vi "LTVDiffDriveCtrl_Execute_TrajState.vi"(5 "LTV_DiffDriveCtrl_Model":T5={"Track Width"=0.2, "Diff_Drive_Linear_System"={"m_A"=[], "m_B"=[], "m_C"=[], "m_D"=[], "States"=0, "Inputs"=0, "Outputs"=0}, "LTV_DiffDriveCtrl_Control"={"Max left vel ctrl effort V"=12.0, "Desired Heading Ctrl Tol Rad"=0.06, "Desired Y Pos Meas Tol M"=0.125, "Desired X Pos Ctrl Tol M"=0.125, "Desired Left Vel Ctrl Tol M/S"=0.1, "Desired Right Vel Ctrl Tol M/S"=0.1, "Max right vel ctrl effort V"=12.0}, "LTV_DiffDriveCtrl_Tolerance"={"Max Heading Tolerance Rad"=0.2, "Max X Tolerance M"=0.0625, "Max Y Tolerance M"=0.125, "Max Left Vel Tol M/S"=0.2, "Max Right Vel Tol M/S"=0.2}, "dT Sec"=0.02} {"LTV_DiffDriveCtrl_Tolerance"."Max Right Vel Tol M/S" format="%#_13g"; "LTV_DiffDriveCtrl_Tolerance"."Max Left Vel Tol M/S" format="%#_13g"; "LTV_DiffDriveCtrl_Tolerance"."Max Y Tolerance M" format="%#_13g"; "LTV_DiffDriveCtrl_Tolerance"."Max X Tolerance M" format="%#_13g"; "LTV_DiffDriveCtrl_Tolerance"."Max Heading Tolerance Rad" format="%#_13g"; "LTV_DiffDriveCtrl_Control"."Max right vel ctrl effort V" format="%#_13g"; "LTV_DiffDriveCtrl_Control"."Desired Right Vel Ctrl Tol M/S" format="%#_13g"; "LTV_DiffDriveCtrl_Control"."Desired Left Vel Ctrl Tol M/S" format="%#_13g"; "LTV_DiffDriveCtrl_Control"."Desired X Pos Ctrl Tol M" format="%#_13g"; "LTV_DiffDriveCtrl_Control"."Desired Y Pos Meas Tol M" format="%#_13g"; "LTV_DiffDriveCtrl_Control"."Desired Heading Ctrl Tol Rad" format="%#_13g"; "LTV_DiffDriveCtrl_Control"."Max left vel ctrl effort V" format="%#_13g"; "Track Width" format="%#_13g"}, 8 "Right Velocity":dbl, 9 "Left Velocity":dbl, 10 "CurrentPose":T2={"TRANSLATION"={"X"=0.0, "Y"=0.0}, "ROTATION"={"VALUE"=0.0, "COS"=1.0, "SIN"=0.0}} {"ROTATION"."SIN" format="%13.4f"; "ROTATION"."COS" format="%13.4f"; "ROTATION"."VALUE" format="%13.4f"; "TRANSLATION"."Y" format="%14.3f"; "TRANSLATION"."X" format="%14.3f"}, 11 "TRAJ_STATE":T1={"TimeSeconds"=0.0, "Velocity"=0.0, "Acceleration"=0.0, "POSE"={"TRANSLATION"={"X"=0.0, "Y"=0.0}, "ROTATION"={"VALUE"=0.0, "COS"=1.0, "SIN"=0.0}}, "Curvature"=0.0} {"POSE"."ROTATION"."SIN" format="%13.4f"; "POSE"."ROTATION"."COS" format="%13.4f"; "POSE"."ROTATION"."VALUE" format="%13.4f"; "POSE"."TRANSLATION"."Y" format="%14.3f"; "POSE"."TRANSLATION"."X" format="%14.3f"}) -> (0 "Error":bool, 1 "At Reference":bool, 2 "Right Motor Dmd":dbl, 3 "Left Motor Dmd":dbl, 4 "out LTV_DiffDrive_CONTROLLER":T10)   [LabVIEW 2019, in "Trajectory_Library.lvlib"]
doc: "The linear time-varying (LTV) differential drive controller has a similar form to the LQR, but the model used to compute the controller gain is the nonlinear model linearized around the drivetrain's current state. We precomputed gains for important places in our state-space, then interpolated between them with a look up table (LUT) to save computational resources.Filters the provided voltages to limit a differential drive's linear and angular acceleration.\n\nThis LabVIEW single call function creates and executes the LTV Diff Drive controller. \n\nThe input linear system is defined as:\n - states\n - left velocity (m/s)\n - right velocity (m/s)\n - inputs\n - left voltage (volts)\n - right voltage(volts)\n - outputs\n - left velocity (m/s)\n - right velocity (m/s)\n\n\n\nInputs:\n - LTVDiffDriveCtrl Model -- cluster -- Packed data used to construct the LTV Diff Drive control system.\n - Traj state -- Traj state -- The desired trajectory state. Contains desired position and velocity values. (Meters, radians)\n - Ref Left Velocity -- double -- The desired left velocity (Meters/sec)\n - Ref Right Velocity -- double -- The desired right velocity (Meters/sec)\n - Current Pose -- Pose2d -- The current pose. (Meters, Radians)\n - Left Velocity -- double -- The current left velocity (Meters/sec)\n - Right Velocity -- double -- The current right velocity (Meters/sec)\n\nOutputs:\n - Left Motor Dmd -- double -- Left wheel motor demand (+/- 1.0)\n - Right Motor Dmd -- double -- Left wheel motor demand (+/- 1.0)\n - At Reference -- boolean -- If TRUE, the current position is within the tolerance.\n - Error -- boolean -- If TRUE, an error occured.\n - out LTV DiffDriveCtrl -- cluster -- Internal data structure."
uses:
  Trajectory_Library.lvlib
  TypeDef/LTV_DIFF_DRIVE_CTRL.ctl
  TypeDef/FUNCTION_GENERATOR_MATRIX.ctl
  <vilib>/Analysis/Matrix/Datatypes/RealMatrix.ctl
  TypeDef/POSE2D.ctl
  TypeDef/TRANSLATION2D.ctl
  TypeDef/ROTATION2D.ctl
  TypeDef/LTV_DIFF_DRIVE_CTRL_MODEL_PARAMS.CTL
  TypeDef/LINEAR_SYSTEM.ctl
  TypeDef/LTV_DIFF_DRIVE_CTRL_CONTROL_PARAMS.CTL
  TypeDef/LTV_DIFF_DRIVE_CTRL_TOLERANCE.CTL
  TypeDef/TRAJ_STATE.ctl
  <vilib>/Analysis/Matrix/NI_Matrix.lvlib
panel:
  # "<States,States>"
  # "<States,Inputs>"
  # "<Outputs,States>"
  # "<Outputs,Inputs>"
  # "< 5, 1 >"
  # "< 2, 1 >"
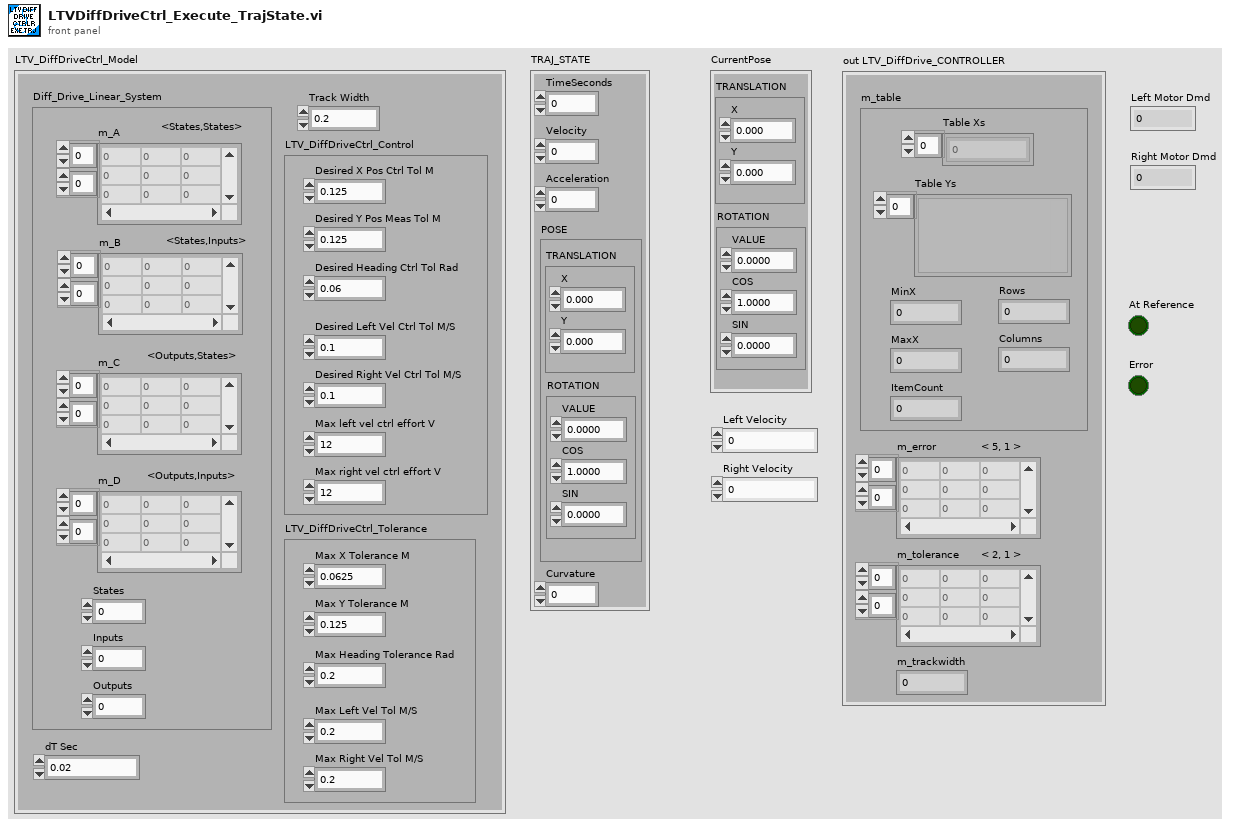
[diagram p1: front panel]
types:
  T1 = typedef "Trajectory_Library.lvlib/TRAJ_STATE.ctl" = cluster{"TimeSeconds":dbl, "Velocity":dbl, "Acceleration":dbl, "POSE":T2, "Curvature":dbl}
  T2 = typedef "Trajectory_Library.lvlib/POSE2D.ctl" = cluster{"TRANSLATION":T3, "ROTATION":T4}
  T3 = typedef "Trajectory_Library.lvlib/TRANSLATION2D.ctl" = cluster{"X":dbl, "Y":dbl}
  T4 = typedef "Trajectory_Library.lvlib/ROTATION2D.ctl" = cluster{"VALUE":dbl, "COS":dbl, "SIN":dbl}
  T5 = typedef "Trajectory_Library.lvlib/LTV_DIFF_DRIVE_CTRL_MODEL_PARAMS.CTL" = cluster{"Track Width":dbl, "Diff_Drive_Linear_System":T6, "LTV_DiffDriveCtrl_Control":T8, "LTV_DiffDriveCtrl_Tolerance":T9, "dT Sec":dbl}
  T6 = typedef "Trajectory_Library.lvlib/LINEAR_SYSTEM.ctl" = cluster{"m_A":T7, "m_B":T7, "m_C":T7, "m_D":T7, "States":i32, "Inputs":i32, "Outputs":i32}
  T7 = typedef "NI_Matrix.lvlib/RealMatrix.ctl" = dbl[][]
  T8 = typedef "Trajectory_Library.lvlib/LTV_DIFF_DRIVE_CTRL_CONTROL_PARAMS.CTL" = cluster{"Max left vel ctrl effort V":dbl, "Desired Heading Ctrl Tol Rad":dbl, "Desired Y Pos Meas Tol M":dbl, "Desired X Pos Ctrl Tol M":dbl, "Desired Left Vel Ctrl Tol M/S":dbl, "Desired Right Vel Ctrl Tol M/S":dbl, "Max right vel ctrl effort V":dbl}
  T9 = typedef "Trajectory_Library.lvlib/LTV_DIFF_DRIVE_CTRL_TOLERANCE.CTL" = cluster{"Max Heading Tolerance Rad":dbl, "Max X Tolerance M":dbl, "Max Y Tolerance M":dbl, "Max Left Vel Tol M/S":dbl, "Max Right Vel Tol M/S":dbl}
  T10 = typedef "Trajectory_Library.lvlib/LTV_DIFF_DRIVE_CTRL.ctl" = cluster{"m_table":T11, "m_error":T7, "m_tolerance":T7, "m_trackwidth":dbl}
  T11 = typedef "Trajectory_Library.lvlib/FUNCTION_GENERATOR_MATRIX.ctl" = cluster{"Table Xs":dbl[], "Table Ys":variant[], "MinX":dbl, "MaxX":dbl, "ItemCount":i32, "Rows":i32, "Columns":i32}
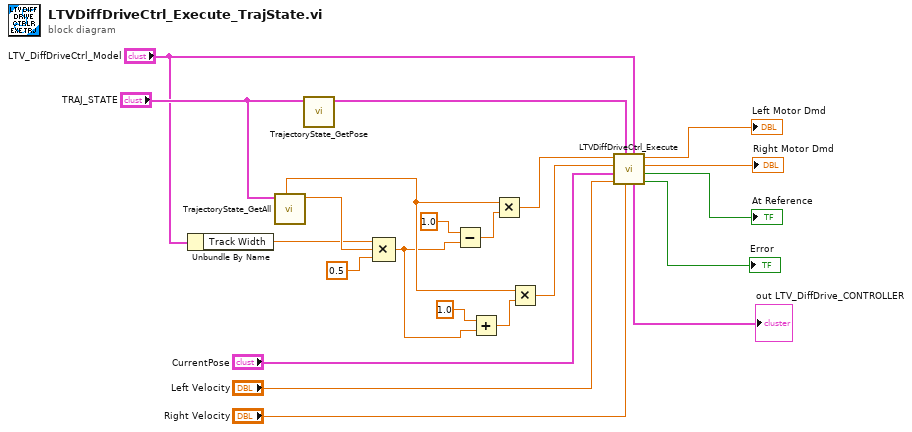
[diagram p0: block diagram]
diagram:
  n1 = Unbundle By Name("LTV_DiffDriveCtrl_Model") -> ("Track Width"=w3:dbl)
  n2 = call "TrajectoryState_GetAll.vi"("TRAJ_STATE"="TRAJ_STATE") -> ("Curvature"=w11:dbl, "Velocity"=w7:dbl)  [unwired: 4 in, 5 out]
  n3 = call "TrajectoryState_GetPose.vi"("TRAJ_STATE"="TRAJ_STATE") -> ("TrajStatePose"=w22:T2)  [unwired: 10 in]
  n4 = Compound Arithmetic op=MULTIPLY(w3, w11, 0.5 ("value")) -> (w6:dbl)
  n5 = Subtract(x=1.0, y=w6) -> (x-y=w10:dbl)
  n6 = Add(x=1.0, y=w6) -> (x+y=w8:dbl)
  n7 = Multiply(x=w7, y=w10) -> (x*y=w2:dbl)
  n8 = Multiply(x=w7, y=w8) -> (x*y=w1:dbl)
  n9 = call "LTVDiffDriveCtrl_Execute.vi"("LTV_DiffDriveCtrl_Model"="LTV_DiffDriveCtrl_Model", "Right Velocity"="Right Velocity", "RefPose"=w22, "Left Velocity"="Left Velocity", "CurrentPose"="CurrentPose", "Ref Right Velocity"=w1, "Ref Left Velocity"=w2) -> ("Error"=→"Error":bool, "At Reference"=→"At Reference":bool, "Right Motor Dmd"=→"Right Motor Dmd":dbl, "Left Motor Dmd"=→"Left Motor Dmd":dbl, "out LTV_DiffDrive_CONTROLLER"=→"out LTV_DiffDrive_CONTROLLER":T10)
